vi "Initilize Streaming.vi"(8 "error in (no error)":errorcluster, 11 "DAQ_msgHandler StreamTypeDef":T1) -> (0 "error out":errorcluster, 3 "DAQ_msgHandler StreamTypeDef 2":T1)   [LabVIEW 2024]
doc: "This VI uses the TDMS Write function to write data to a TDMS file."
uses:
  controls/DAQ_msgHandler StreamTypeDef.ctl
  CTRsample/Control/streamIO_states.ctl
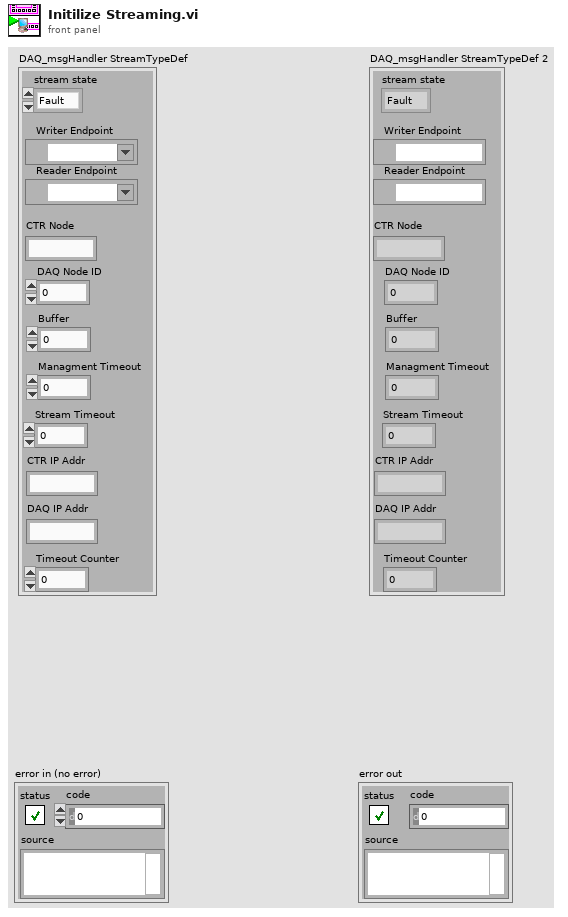
[diagram p1: front panel]
types:
  T1 = typedef "DAQ_msgHandler StreamTypeDef.ctl" = cluster{"stream state":T2, "CTR Node":string, "DAQ Node ID":i32, "Writer Endpoint":refnum<k21>, "Reader Endpoint":refnum<k21>, "Buffer":i32, "Managment Timeout":i32, "Stream Timeout":i32, "DAQ IP Addr":string, "CTR IP Addr":string, "Timeout Counter":i32}
  T2 = typedef "streamIO_states.ctl" = enum16{"Fault", "Initialize", "Stream", "Close"}
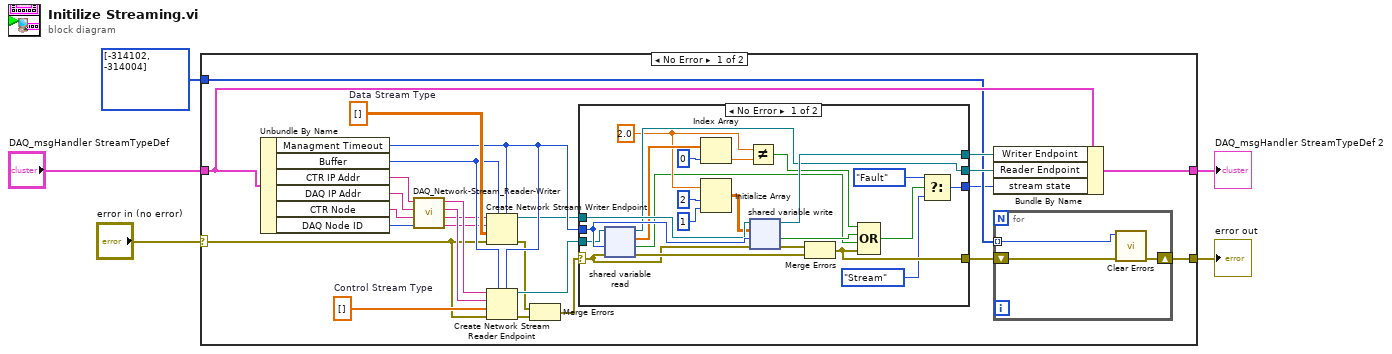
[diagram p0: block diagram]
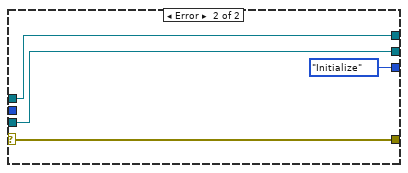
[diagram p2: hidden frame]
diagram:
  n1 = case shown="No Error" "error in (no error)" {
    selector: "error in (no error)" -> [w17 w63]
    tunnel: [w12 w63] -> w5
    tunnel: "DAQ_msgHandler StreamTypeDef" -> [w31 w62]
    tunnel: [w30 w62] -> w2
    tunnel: i32[] [-314102, -314004] -> [w9 _]
    frame No Error {
      w29 = dbl[][] []  # Data Stream Type
      w28 = dbl[] []  # Control Stream Type
      n2 = Unbundle By Name(w31) -> ("Managment Timeout"=w27:i32, "Buffer"=w26:i32, "CTR IP Addr"=w14:string, "DAQ IP Addr"=w13:string, "CTR Node"=w15:string, "DAQ Node ID"=w16:i32)
      n3 = call "DAQ_Network-Stream_Reader-Writer.vi"("DAQ ID"=w16, "CTR Endpoint"=w15, "DAQ IP Addr"=w13, "CTR IP Addr"=w14) -> ("//CTR IP Addr:CTR000/DAQ000-Data"=w18:string, "//DAQ IP Addr:DAQ000/DAQ000-Data"=w19:string, "//CTR IP Addr:CTR000/DAQ000-Control"=w20:string, "//DAQ IP Addr:DAQ000/DAQ000-Control"=w21:string)  [unwired: 4 in]
      n4 = Create Network Stream Writer Endpoint(5:w27, 7:w26, 8:w17, 9:w29, 10:w18, 11:w19) -> (0:w10:errorcluster, 3:w24:refnum<k21>)  [unwired: 1 in]
      n5 = Create Network Stream Reader Endpoint(5:w27, 7:w26, 8:w17, 9:w28, 10:w20, 11:w21) -> (0:w11:errorcluster, 3:w25:refnum<k21>)  [unwired: 1 in]
      n6 = Merge Errors(w10, w11) -> (w8:errorcluster)
      n7 = case shown="No Error" w8 {
        selector: w8 -> [w44 w58]
        tunnel: w27 -> [w54 _]
        tunnel: w25 -> [w53 w57]
        tunnel: w24 -> [w52 w56]
        tunnel: [w51 w56] -> w23
        tunnel: [w50 w57] -> w22
        tunnel: [w47 w58] -> w7
        tunnel: [w32 streamIO_states."Initialize" ("stream state")] -> w6
        frame No Error {
          w40 = 2.0
          n8 = shared-variable-read(w53, w44, w54) -> (w50:refnum<k21>, w49:errorcluster, w33:bool, w45:dbl[])
          n9 = Index Array(array=w45, index=0) -> (element=w37:dbl)
          n10 = Initialize Array(w40, 2 ("dimension size"), 1 ("dimension size")) -> (w41:dbl[][])
          n11 = Not Equal?(x=w40, y=w37) -> (x != y?=w39:bool)
          n12 = shared-variable-write(w52, w44, w41, w54) -> (w51:refnum<k21>, w48:errorcluster, w34:bool)
          n13 = Merge Errors(w48, w49) -> (w47:errorcluster)
          n14 = Compound Arithmetic op=OR(w39, w34, w33, w47) -> (w38:bool)
          n15 = Select(t=streamIO_states."Fault" ("stream state"), s=w38, f=streamIO_states."Stream" ("stream state")) -> (s? t:f=w32:T2)
        }
        frame Error {
        }
      }
      n16 = Bundle By Name(cluster=w31, "Writer Endpoint"=w23, "Reader Endpoint"=w22, "stream state"=w6) -> (w30:T1)
      n17 = for {
        shift-right: [w60] -> w12
        shift-left: w7 -> [w61]
        tunnel: w9 -> [w59] mode=indexing
        n18 = call <vilib>:"Clear Errors.vi"("error in (no error)"=w61, "specific error code to clear (0: all)"=w59) -> ("error out"=w60:errorcluster)  [unwired: 4 in, 1 out]
      }
    }
    frame Error {
    }
  }
  "error out" <- w5
  "DAQ_msgHandler StreamTypeDef 2" <- w2
